vi "PUSH DB strings DISPLAY.vi"(6 "CLEAR LIST?":bool, 8 "error in (no error)":errorcluster, 10 "NEW String":string) -> (0 "error out":errorcluster)   [LabVIEW 2020]
uses:
  <vilib>/Rock Robotics/Network Tables/NT Read String.vi
  <vilib>/Rock Robotics/Network Tables/NT Write String.vi
panel:
  out "subarray":string[](array[string])
  out "appended array":string[](array[string])
  out "DB string read":string[](array[string])
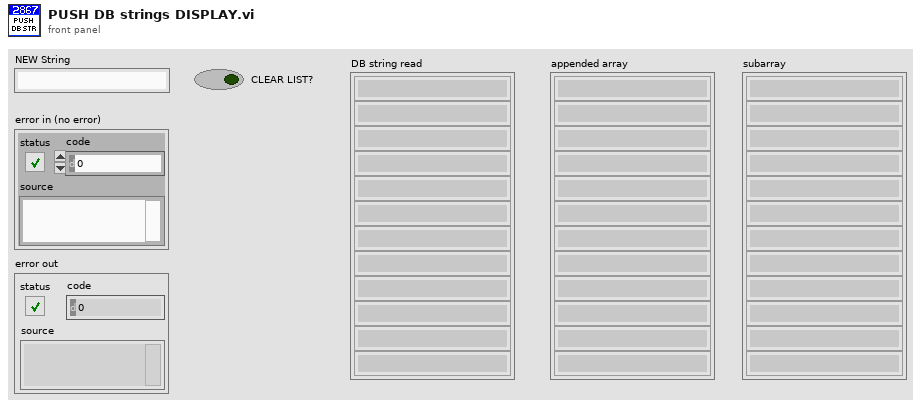
[diagram p1: front panel]
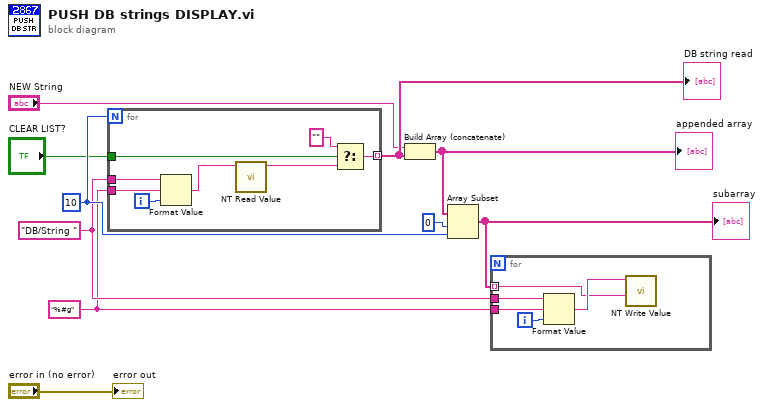
[diagram p0: block diagram]
diagram:
  w3 = "%#g" ("format string")
  w4 = "DB/String "
  w6 = 10
  n1 = for {
    N: w6 -> [_]
    tunnel: w4 -> [w18]
    tunnel: w3 -> [w17]
    tunnel: [w14] -> w10 mode=indexing
    tunnel: "CLEAR LIST?" -> [w11]
    i -> [w16]
    n2 = Format Value(string ("")=w18, format string=w17, value (0)=w16) -> (output string=w15:string)
    n3 = call-poly <vilib>:"NT Read Value.vi"("Name"=w15) -> ("String"=w13:string)  [unwired: 9 in, 1 out]
    n4 = Select(t="", s=w11, f=w13) -> (s? t:f=w14:string)
  }
  "DB string read" <- w10
  n5 = Build Array (concatenate)("NEW String", w10) -> (w8:string[])
  "appended array" <- w8
  n6 = Array Subset(array=w8, index=0, length=w6) -> (w5:string[])
  "subarray" <- w5
  n7 = for {
    tunnel: w4 -> [w23]
    tunnel: w3 -> [w22]
    tunnel: w5 -> [w19] mode=indexing
    i -> [w21]
    n8 = Format Value(string ("")=w23, format string=w22, value (0)=w21) -> (output string=w20:string)
    n9 = call-poly <vilib>:"NT Write Value.vi"("String"=w19, "Name"=w20) -> ()  [unwired: 9 in, 1 out]
  }
  "error out" <- "error in (no error)"
